vi "UI change exposure time.vi"(8 "error in (no error)":errorcluster, 10 "exposure time":dbl, 11 "Main_Control in":refnum<class "Main_Control.lvclass">) -> (0 "error out":errorcluster, 3 "Main_Control out":refnum<class "Main_Control.lvclass">)   [LabVIEW 2021, in "Main_Control.lvlib" / "Main_Control.lvclass"]
uses:
  Main_Control.lvclass
  Main_Control.lvclass/Main_Control.ctl
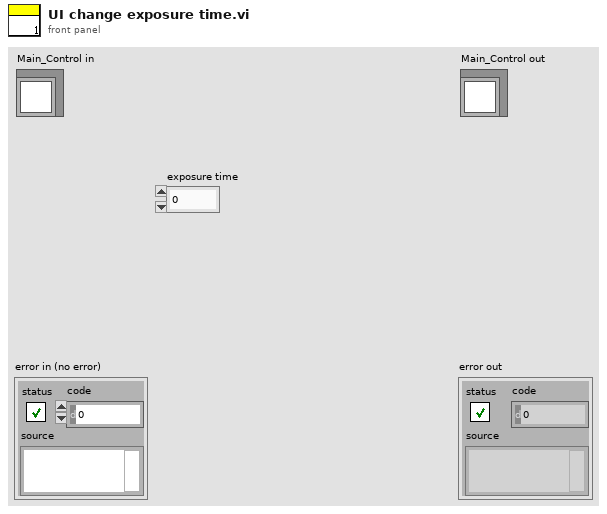
[diagram p1: front panel]
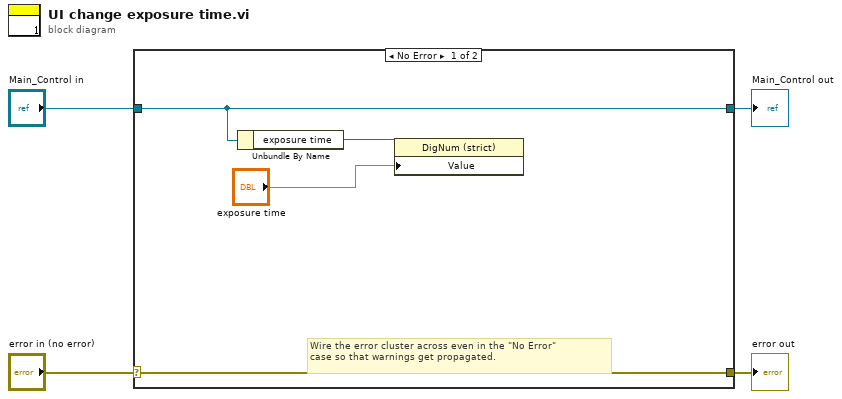
[diagram p0: block diagram]
diagram:
  n1 = case shown="No Error" "error in (no error)" {
    selector: "error in (no error)" -> [w8 w10]
    tunnel: [w8 w10] -> w3
    tunnel: [w7 w9] -> w1
    tunnel: "Main_Control in" -> [w7 w9]
    frame No Error {
      # "Wire the error cluster across even in the \"No Error\"\ncase so that warnings get propagated."
      n2 = Unbundle By Name(w7) -> ("exposure time"=w6:refnum<vi>)
      n3 = property class="DigNum (strict)"(reference=w6, "Value"="exposure time") -> ()  [unwired: 1 in, 2 out]
    }
    frame Error {
    }
  }
  "error out" <- w3
  "Main_Control out" <- w1
